vi "LVObject to JSON.vi"(5 "enable LabVIEW extensions? (T)":bool=TRUE, 6 "Pretty Print?":bool, 7 "JSONtext LVClass Serializer in":refnum<class "JSONtext LVClass Serializer.lvclass">, 8 "error in (no error)":errorcluster, 10 "Object":refnum<class>) -> (0 "error out":errorcluster, 2 "<JSON>Object":string)   [LabVIEW 2019, in "JSONtext LVClass Serializer.lvclass"]
doc: "Convert Object of a LabVIEW Class to a JSON representation."
uses:
  JSONtext LVClass Serializer.lvclass
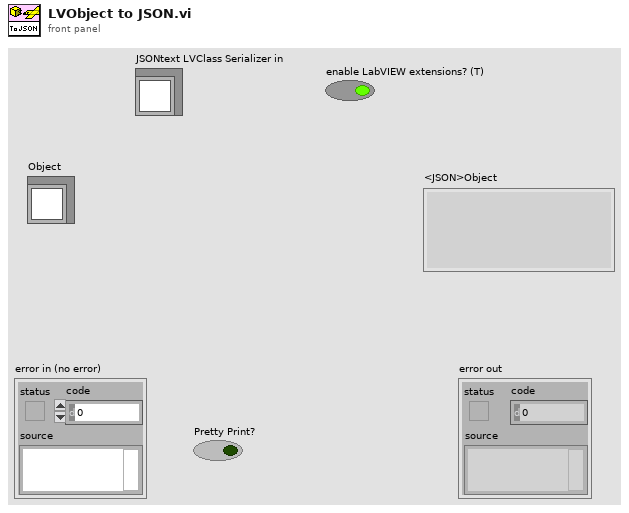
[diagram p1: front panel]
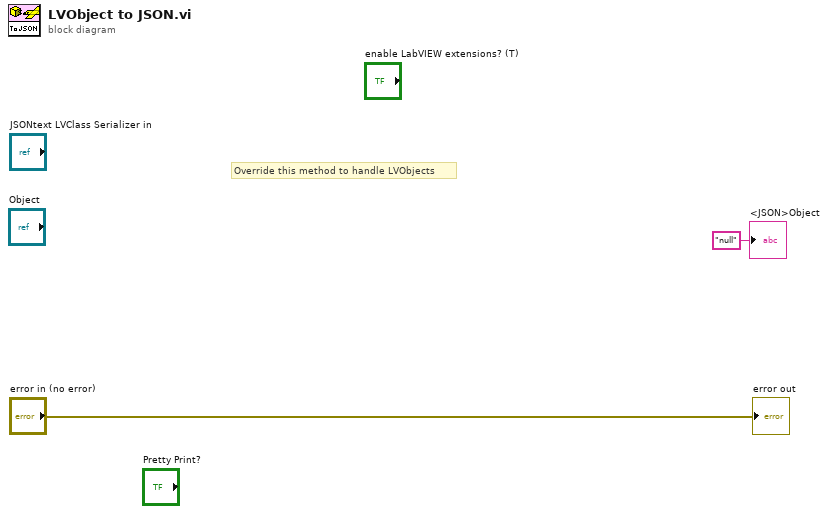
[diagram p0: block diagram]
diagram:
  # "Override this method to handle LVObjects"
  "error out" <- "error in (no error)"
  "<JSON>Object" <- "null" ("<JSON>Object")
